vi "Calculate Stats Rectangles.vi"(9 "Start y":i32, 10 "Start x":i32, 11 "Count":i32) -> (3 "Rectangles":T1[](array[typedef]))   [LabVIEW 2021, in "Ship.lvclass"]
uses:
  Ship.lvclass
  LabSDL2/Source/Libraries/LibSDL2 Wrapper/Controls/Rectangle.ctl
  LabSDL2/Source/Libraries/LibSDL2 Wrapper/LibSDL2.lvlib
panel:
  in  "Width":i32=6
  in  "Spacing":i32=3
  in  "Height":i32=4
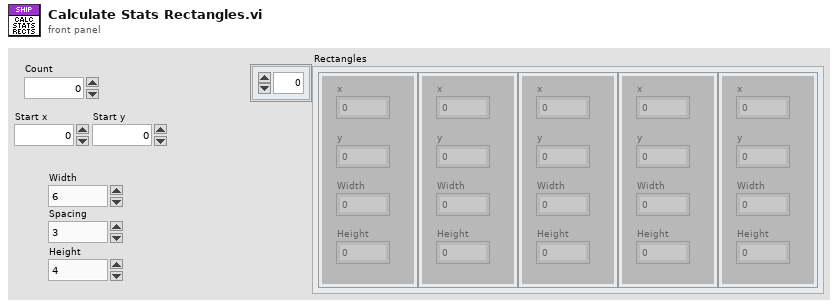
[diagram p1: front panel]
types:
  T1 = typedef "LibSDL2.lvlib/Rectangle.ctl" = cluster{"x":i32, "y":i32, "Width":i32, "Height":i32}
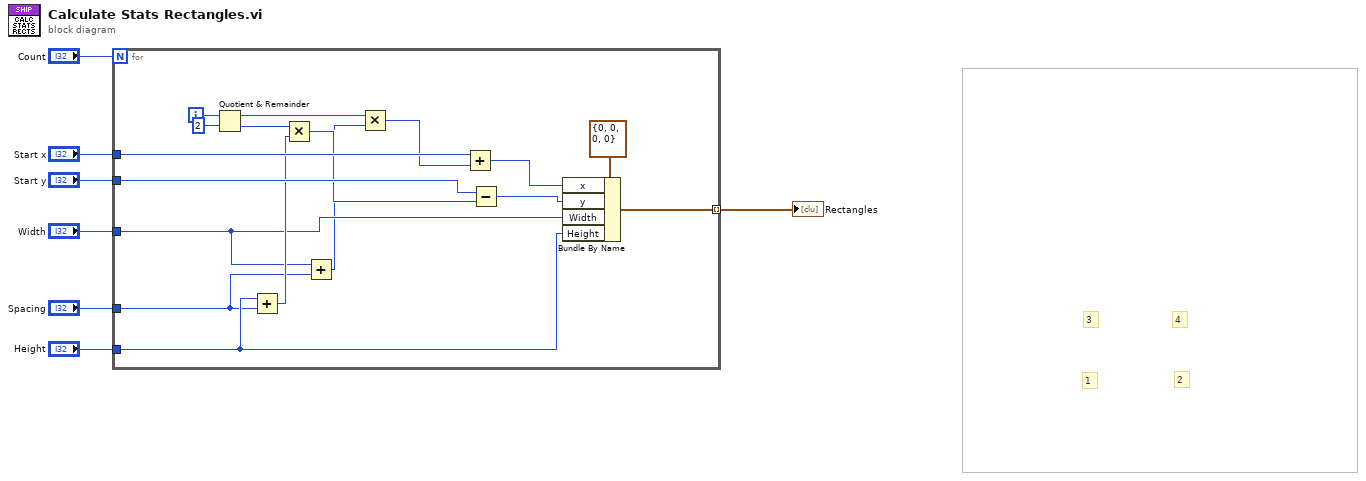
[diagram p0: block diagram]
diagram:
  # "4"
  # "3"
  # "2"
  # "1"
  n1 = for {
    N: "Count" -> [_]
    tunnel: [w21] -> w7 mode=indexing
    tunnel: "Start x" -> [w19]
    tunnel: "Spacing" -> [w11]
    tunnel: "Width" -> [w12]
    tunnel: "Height" -> [w15]
    tunnel: "Start y" -> [w17]
    i -> [w23]
    n2 = Quotient & Remainder(x=w23, y=2) -> (x-y*floor(x/y)=w10:i32, floor(x/y)=w16:i32)
    n3 = Add(x=w15, y=w11) -> (x+y=w14:i32)
    n4 = Multiply(x=w16, y=w14) -> (x*y=w13:i32)
    n5 = Add(x=w12, y=w11) -> (x+y=w9:i32)
    n6 = Multiply(x=w10, y=w9) -> (x*y=w8:i32)
    n7 = Add(x=w19, y=w8) -> (x+y=w20:i32)
    n8 = Subtract(x=w17, y=w13) -> (x-y=w18:i32)
    n9 = Bundle By Name(cluster=T1 {"x"=0, "y"=0, "Width"=0, "Height"=0} ("Rectangle"), "x"=w20, "y"=w18, "Width"=w12, "Height"=w15) -> (w21:T1)
  }
  "Rectangles" <- w7
